vi "采样延时设置.vi"(8 "错误输入（无错误）":errorcluster, 10 "NewVal":i32, 11 "VISA引用句柄输入":refnum<visa-resource-name>) -> (0 "error out":errorcluster caption="错误输出", 3 "读取缓冲区":string)   [LabVIEW 2017]
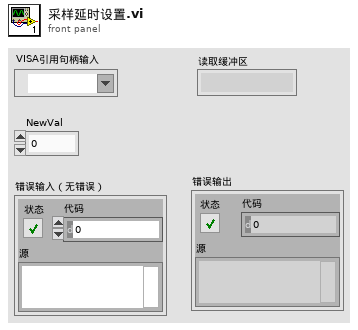
[diagram p1: front panel]
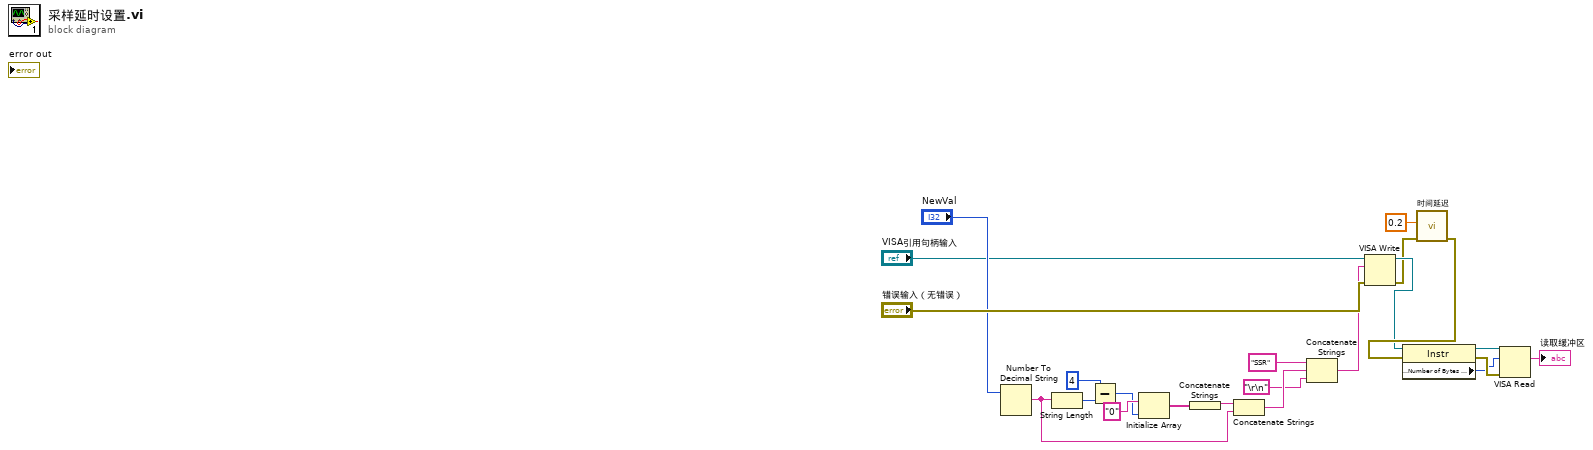
[diagram p0: block diagram]
diagram:
  n1 = Number To Decimal String(number="NewVal") -> (decimal integer string=w11:string)  [unwired: 1 in]
  n2 = String Length(string=w11) -> (length=w5:i32)
  n3 = Subtract(x=4, y=w5) -> (x-y=w7:i32)
  n4 = Initialize Array("0", w7) -> (w9:string[])
  n5 = Concatenate Strings(w9) -> (w10:string)
  n6 = Concatenate Strings(w10, w11) -> (w12:string)
  n7 = Concatenate Strings("SSR" ("写入缓冲区"), w12, "\r\n") -> (w13:string)
  n8 = VISA Write(VISA resource name="VISA引用句柄输入", write buffer=w13, error in (no error)="错误输入（无错误）") -> (VISA resource name out=w20:refnum<visa-resource-name>, error out=w15:errorcluster)  [unwired: 1 out]
  n9 = call "时间延迟"("error in (no error)"=w15, "Delay Time (s)"=0.2) -> ("error out"=w21:errorcluster)  [unwired: 9 in]
  n10 = property class="Instr"(reference=w20, error in=w21) -> (reference out=w19:refnum<visa-resource-name>, error out=w18:errorcluster, "Serial Settings:Number of Bytes at Serial Port"=w17:u32)
  n11 = VISA Read(VISA resource name=w19, byte count=w17, error in (no error)=w18) -> (read buffer=→"读取缓冲区":string)  [unwired: 3 out]
